vi "class_data.vi"() -> ()   [LabVIEW 2010, in "CPUmonitor.lvclass"]
uses:
  CPUmonitor.lvclass
panel:
  in  "exit?":bool
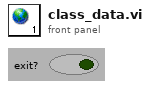
[diagram p1: front panel]
diagram:
